vi "FormatDMAelement_10_elements_with_scale.vi"(8 "valid in":bool, 10 "factor":u16, 11 "Data in":fxp<+/-,32,14>[](array[numeric])=[0.0, 0.0, 0.0, 0.0, 0.0, 0.0, 0.0, 0.0, 0.0, 0.0]) -> (0 "valid out":bool, 3 "Values":u64[](array[numeric]))   [LabVIEW 2018]
uses:
  <vilib>/rvi/FXPMathLib/FxpInterpret/XNode/nifxpmath_Interpret.xnode
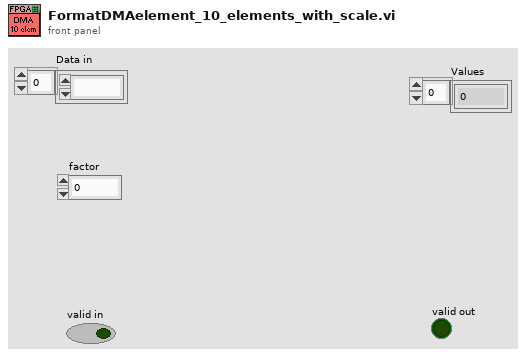
[diagram p1: front panel]
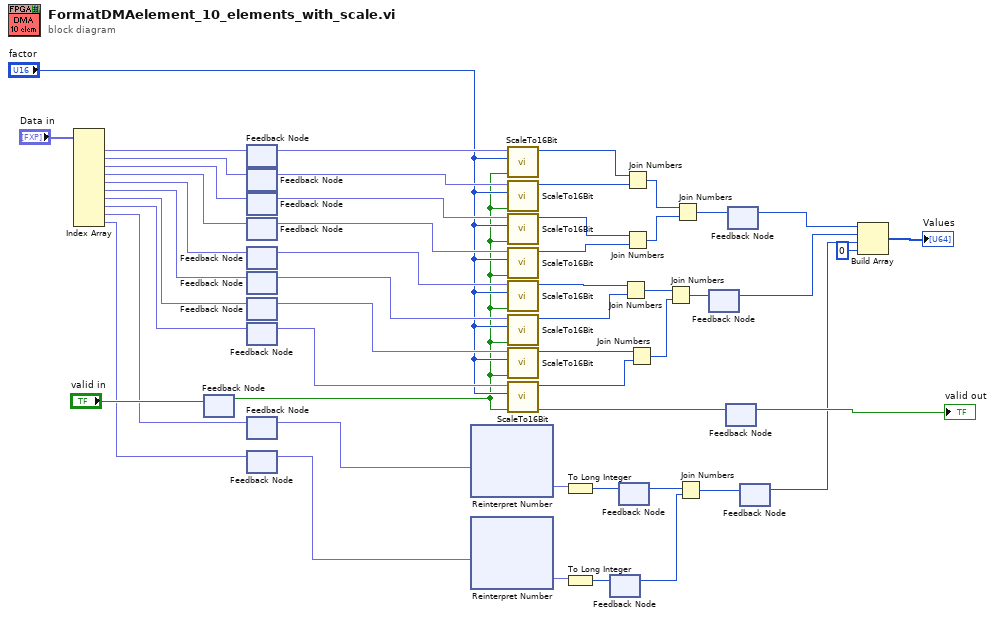
[diagram p0: block diagram]
diagram:
  n1 = Index Array(array="Data in") -> (element #1=w50:fxp<+/-,32,14>, element #2=w49:fxp<+/-,32,14>, element #3=w48:fxp<+/-,32,14>, element #4=w47:fxp<+/-,32,14>, element #5=w44:fxp<+/-,32,14>, element #6=w43:fxp<+/-,32,14>, element #7=w34:fxp<+/-,32,14>, element #8=w33:fxp<+/-,32,14>, element #9=w13:fxp<+/-,32,14>, element #10=w12:fxp<+/-,32,14>)  [unwired: 10 in]
  n2 = feedback #1() -> (w23:bool)  [unwired: 1 in]
  n3 = feedback-in #1("valid in") -> ()
  n4 = feedback #2() -> (w32:fxp<+/-,32,14>)  [unwired: 1 in]
  n5 = feedback-in #2(w50) -> ()
  n6 = feedback #3() -> (w31:fxp<+/-,32,14>)  [unwired: 1 in]
  n7 = feedback-in #3(w49) -> ()
  n8 = feedback #4() -> (w30:fxp<+/-,32,14>)  [unwired: 1 in]
  n9 = feedback-in #4(w48) -> ()
  n10 = feedback #5() -> (w29:fxp<+/-,32,14>)  [unwired: 1 in]
  n11 = feedback-in #5(w47) -> ()
  n12 = feedback #6() -> (w28:fxp<+/-,32,14>)  [unwired: 1 in]
  n13 = feedback-in #6(w44) -> ()
  n14 = feedback #7() -> (w27:fxp<+/-,32,14>)  [unwired: 1 in]
  n15 = feedback-in #7(w43) -> ()
  n16 = feedback #8() -> (w26:fxp<+/-,32,14>)  [unwired: 1 in]
  n17 = feedback-in #8(w34) -> ()
  n18 = feedback #9() -> (w25:fxp<+/-,32,14>)  [unwired: 1 in]
  n19 = feedback-in #9(w33) -> ()
  n20 = feedback #10() -> (w10:fxp<+/-,32,14>)  [unwired: 1 in]
  n21 = feedback-in #10(w13) -> ()
  n22 = feedback #11() -> (w8:fxp<+/-,32,14>)  [unwired: 1 in]
  n23 = feedback-in #11(w12) -> ()
  n24 = xnode "Reinterpret Number"("x"=w10) -> ("y"=w11:fxp<+/-,32,32>)
  n25 = xnode "Reinterpret Number"("x"=w8) -> ("y"=w9:fxp<+/-,32,32>)
  n26 = call "ScaleTo16Bit.vi"("valid in"=w23, "factor"="factor", "Value in"=w32) -> ("16bit integer"=w21:i16)  [unwired: 7 in, 1 out]
  n27 = call "ScaleTo16Bit.vi"("valid in"=w23, "factor"="factor", "Value in"=w31) -> ("16bit integer"=w20:i16)  [unwired: 7 in, 1 out]
  n28 = call "ScaleTo16Bit.vi"("valid in"=w23, "factor"="factor", "Value in"=w30) -> ("16bit integer"=w19:i16)  [unwired: 7 in, 1 out]
  n29 = call "ScaleTo16Bit.vi"("valid in"=w23, "factor"="factor", "Value in"=w29) -> ("16bit integer"=w18:i16)  [unwired: 7 in, 1 out]
  n30 = call "ScaleTo16Bit.vi"("valid in"=w23, "factor"="factor", "Value in"=w28) -> ("16bit integer"=w17:i16)  [unwired: 7 in, 1 out]
  n31 = call "ScaleTo16Bit.vi"("valid in"=w23, "factor"="factor", "Value in"=w27) -> ("16bit integer"=w16:i16)  [unwired: 7 in, 1 out]
  n32 = call "ScaleTo16Bit.vi"("valid in"=w23, "factor"="factor", "Value in"=w26) -> ("16bit integer"=w15:i16)  [unwired: 7 in, 1 out]
  n33 = call "ScaleTo16Bit.vi"("valid in"=w23, "factor"="factor", "Value in"=w25) -> ("valid out"=w22:bool, "16bit integer"=w14:i16)  [unwired: 7 in]
  n34 = To Long Integer(number=w11) -> (32bit integer=w6:i32)
  n35 = To Long Integer(number=w9) -> (32bit integer=w7:i32)
  n36 = feedback #12() -> (w4:i32)  [unwired: 1 in]
  n37 = feedback-in #12(w7) -> ()
  n38 = feedback #13() -> (w5:i32)  [unwired: 1 in]
  n39 = feedback-in #13(w6) -> ()
  n40 = Join Numbers(hi=w17, lo=w16) -> ((hi.lo)=w42:u32)
  n41 = Join Numbers(hi=w21, lo=w20) -> ((hi.lo)=w46:u32)
  n42 = Join Numbers(hi=w19, lo=w18) -> ((hi.lo)=w45:u32)
  n43 = Join Numbers(hi=w15, lo=w14) -> ((hi.lo)=w35:u32)
  n44 = Join Numbers(hi=w42, lo=w35) -> ((hi.lo)=w40:u64)
  n45 = Join Numbers(hi=w46, lo=w45) -> ((hi.lo)=w41:u64)
  n46 = Join Numbers(hi=w5, lo=w4) -> ((hi.lo)=w3:u64)
  n47 = feedback #14() -> (w39:u64)  [unwired: 1 in]
  n48 = feedback-in #14(w40) -> ()
  n49 = feedback #15() -> (→"valid out":bool)  [unwired: 1 in]
  n50 = feedback-in #15(w22) -> ()
  n51 = feedback #16() -> (w38:u64)  [unwired: 1 in]
  n52 = feedback-in #16(w41) -> ()
  n53 = feedback #17() -> (w2:u64)  [unwired: 1 in]
  n54 = feedback-in #17(w3) -> ()
  n55 = Build Array(w38, w39, w2, u64 0 ("element")) -> (→"Values":u64[])
